vi "Close.vi"(8 "error in":errorcluster, 11 "Cfg Dev in":refnum<class "PPT.lvclass">) -> (0 "error out":errorcluster, 3 "Cfg Dev out":refnum<class "PPT.lvclass">)   [LabVIEW 2015, in "PPT.lvclass"]
uses:
  PPT.lvclass
  Reusable/Session APIs/Text Communication/Text Device Session.lvclass
  PPT.lvclass/PPT.ctl
  Configurable Device/Configurable Device.lvclass
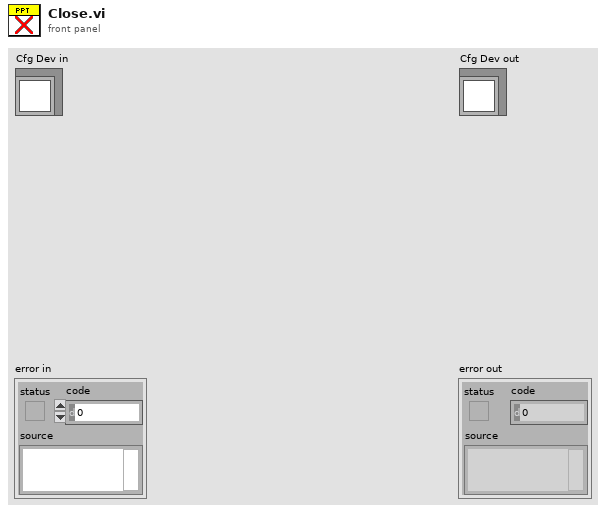
[diagram p1: front panel]
types:
  T1 = typedef "Session - Root.lvclass/Session Handle.ctl" = refnum<data-value>
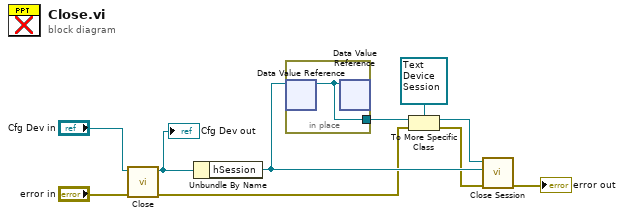
[diagram p0: block diagram]
diagram:
  n1 = call-parent "Close.vi"("error in"="error in", "Cfg Dev in"="Cfg Dev in") -> ("error out"=w2:errorcluster, "Cfg Dev out"=w1:refnum<class "PPT.lvclass">)  [unwired: 8 in]
  "Cfg Dev out" <- w1
  n2 = Unbundle By Name(w1) -> ("hSession"=w10:T1)
  n3 = in-place {
    in-place-border: [w11] -> w9
    n4 = in-place-dvr #1(w10) -> (w11:refnum<class "Session - Root.lvclass">)  [unwired: 1 out]
    n5 = in-place-dvr #1(w11) -> ()  [unwired: 2 out]
  }
  n6 = To More Specific Class(target class=refnum<class "Text Device Session.lvclass"> refnum ("Text Session"), reference=w9, error in=w2) -> (specific class reference=w7:refnum<class "Text Device Session.lvclass">, error out=w5:errorcluster)
  n7 = call-dynamic "Close Session.vi"("error in"=w5, "Session In"=w10, "Text Session"=w7) -> ("error out"=→"error out":errorcluster)  [unwired: 7 in, 1 out]
